vi "Initialize.vi"(6 "optional":variant, 8 "error in":errorcluster, 11 "I64 in":refnum<class "I64.lvclass">) -> (0 "error out":errorcluster, 3 "Node*":refnum<data-value>)   [LabVIEW 2013, in "I64.lvclass"]
doc: "Initializes a node. Makes a data value reference of the node, sets the selfNode, and output the data value reference."
uses:
  I64.lvclass
  xCE/xceNode/xceNode.lvclass
  Channel/Channel.lvclass
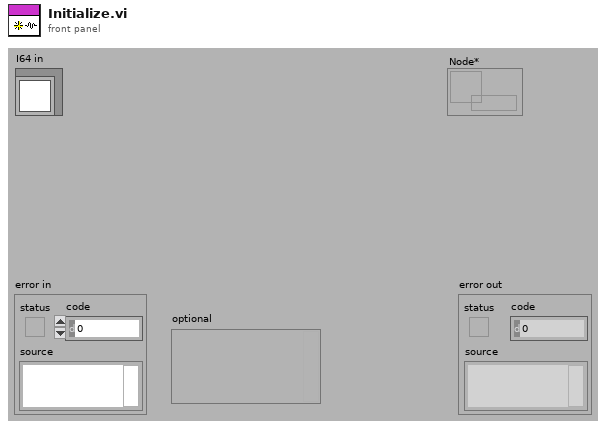
[diagram p1: front panel]
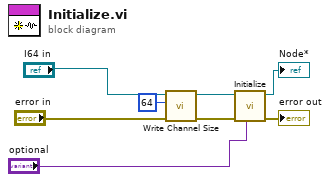
[diagram p0: block diagram]
diagram:
  n1 = call "Write Channel Size.vi"("error in (no error)"="error in", "Channel Size"=64, "Channel in"="I64 in") -> ("error out"=w2:errorcluster, "Channel out"=w3:refnum<class "I64.lvclass">)  [unwired: 7 in]
  n2 = call-parent "Initialize.vi"("optional"="optional", "error in"=w2, "Channel in"=w3) -> ("error out"=→"error out":errorcluster, "Node*"=→"Node*":refnum<data-value>)  [unwired: 7 in]
